vi "Graph_Display.vi"(0 "Data In":T5, 2 "Display State In":T3 {"Time_data" format="%<%.3X>T"}, 3 "Container State":T4) -> (6 "Data Out":T5, 7 "Display State Out":T3 {"Time_data" format="%<%.3X>T"}, 8 "Action":T2)   [LabVIEW 2013, in "2D Buffer Display.xctl"]
doc: "This is the actual display that the user will see when they place the X control on the interface. This display (facade) VI handles user events such as data input and display state changes (i.e. when a control property is updated) as well as an events associated with the actual interface itself (such as scale changes). \nThe 2-D buffer will display a single variable for 0 to n channels where n is specified by the owner of the control. Data in the buffer can be retrieved using properrty nodes as necessary and the amount of data stored in the properrty node can be also adjusted through property nodes."
uses:
  2D Buffer Display.xctl
  Graph_Data.ctl
  <vilib>/_xctls/Container State.ctl
  Graph_State.ctl
  <vilib>/_xctls/Action.ctl
  <vilib>/_xctls/XControlSupport.lvlib
  <vilib>/Analysis/NI_AALBase.lvlib
panel:
  out "Chart":T1(graph)
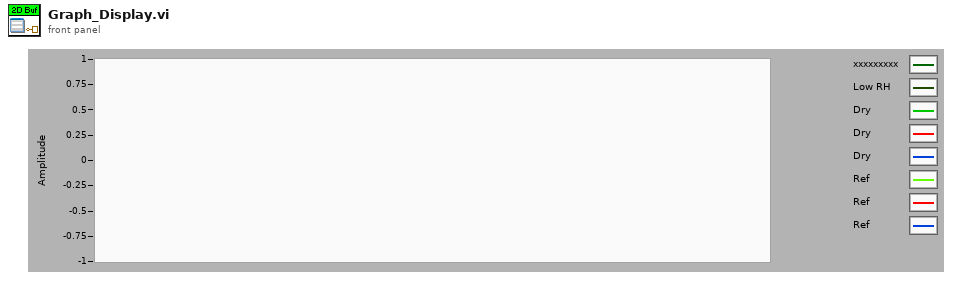
[diagram p1: front panel]
types:
  T1 = cluster{"Time_data":timestamp[], "data_out":sgl[]}[]
  T2 = typedef "XControlSupport.lvlib/Action.ctl" = cluster{"Data Changed?":bool, "State Changed?":bool, "Action Name":string}
  T3 = typedef "2D Buffer Display.xctl/Graph_State.ctl" = cluster{"History":u16, "Time_data":timestamp[], "Data_Out":sgl[][][], "Channels":bool[], "Variable":bool[], "Variable Tags":string[], "Channel Tags":string[], "Plot Details":cluster{"Name":string, "Line Width":u8, "Line Style":u8, "Color":u32}[], "Y-Axis Labels":string[], "Avg Data":cluster{"mean":dbl, "standard deviation":dbl}[][]}
  T4 = typedef "XControlSupport.lvlib/Container State.ctl" = cluster{"Indicator?":bool, "Run Mode?":bool, " Refnum":refnum<vi>}
  T5 = typedef "2D Buffer Display.xctl/Graph_Data.ctl" = cluster{"data_out":sgl[][], "time":timestamp}
  T6 = typedef "LVCursorListTypeDef.ctl" = cluster{"Name":string, "Color":u32, "Style":u8, "Point Style":u8, "Name Visible":bool, "Allow Drag":bool, "Cursor Mode":u32, "Plot":i32, "Index":i32, "Position":cluster{"X":dbl, "Y":dbl}, "X Scale":u32, "Y Scale":u32, "Watch Plots":i32[], "Watch All Plots":bool, "Plot Area":i32, "Label Offset":cluster{"X":dbl, "Y":dbl}}[]
  T7 = cluster{"Name":string, "Line Width":u8, "Line Style":u8, "Color":u32}[]
  T8 = cluster{"Name":string, "Line Width":u8, "Line Style":u8, "Color":u32}
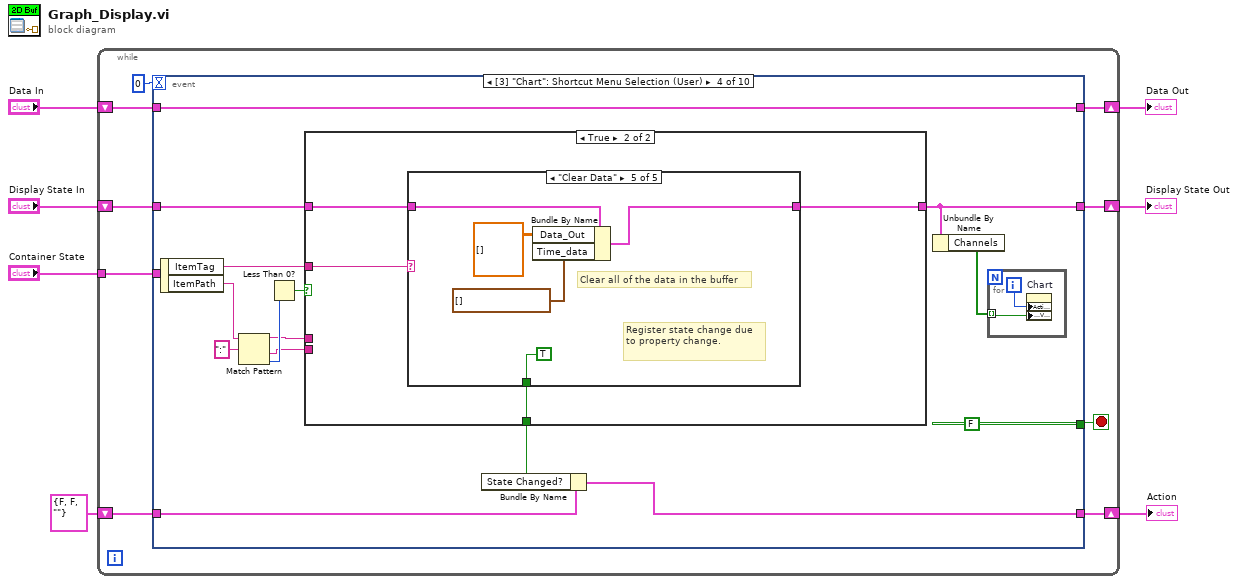
[diagram p0: block diagram]
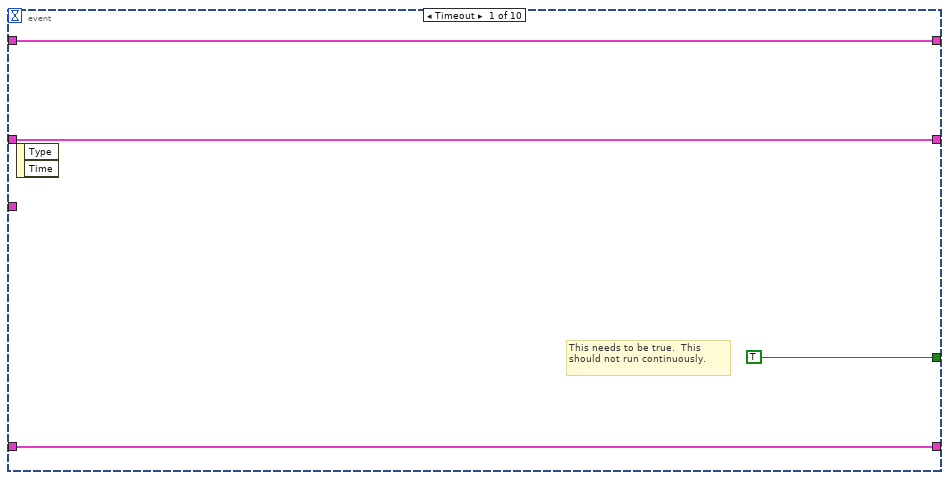
[diagram p2: hidden frame]
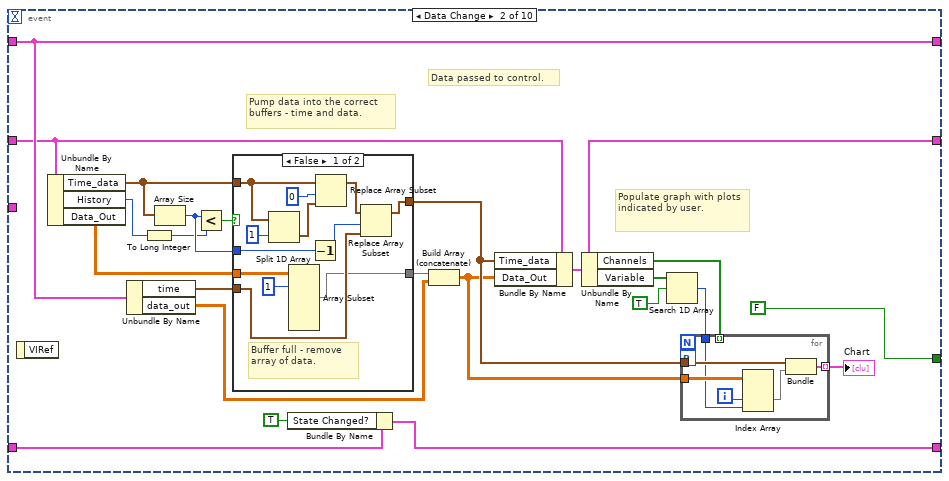
[diagram p3: hidden frame]
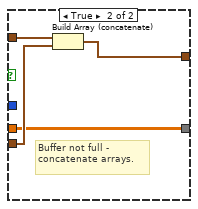
[diagram p4: hidden frame]
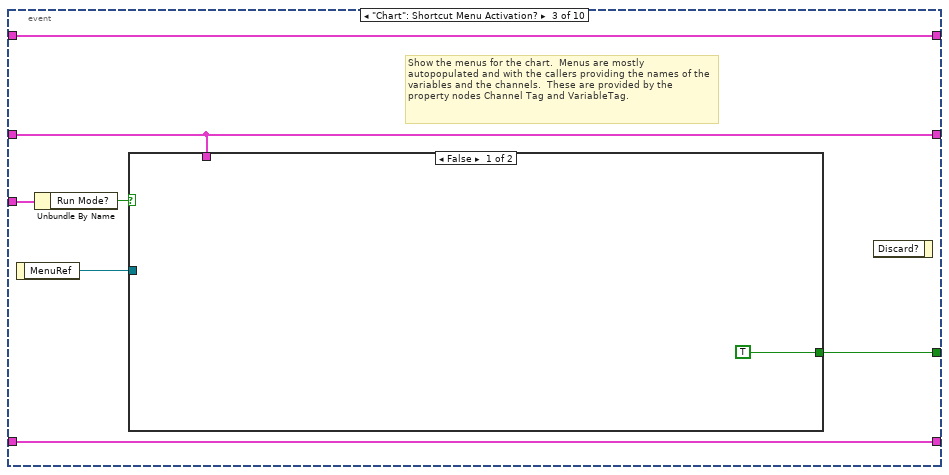
[diagram p5: hidden frame]
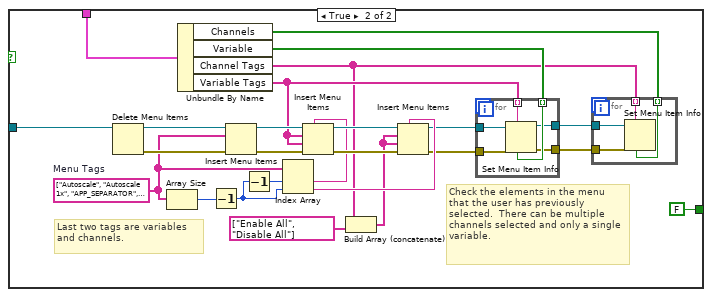
[diagram p6: hidden frame]
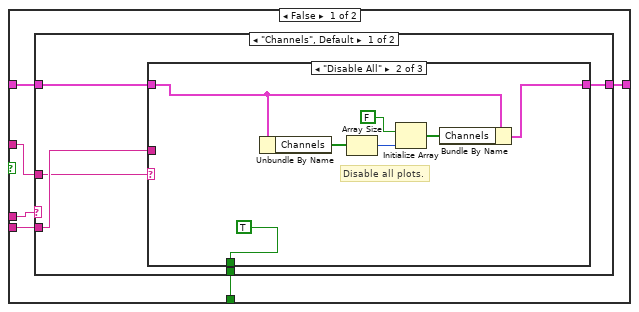
[diagram p7: hidden frame]
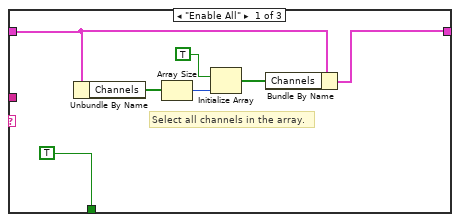
[diagram p8: hidden frame]
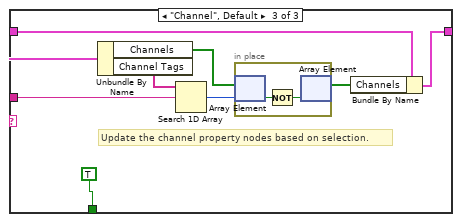
[diagram p9: hidden frame]
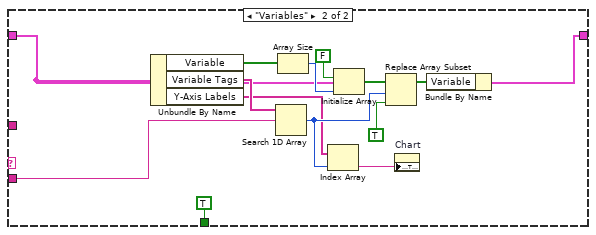
[diagram p10: hidden frame]
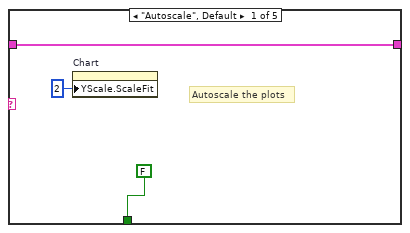
[diagram p11: hidden frame]
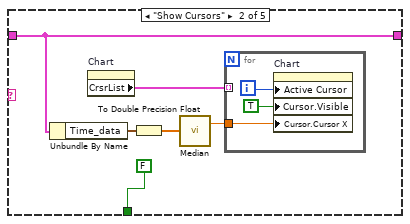
[diagram p12: hidden frame]
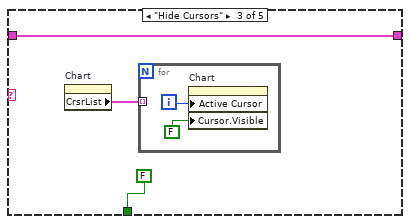
[diagram p13: hidden frame]
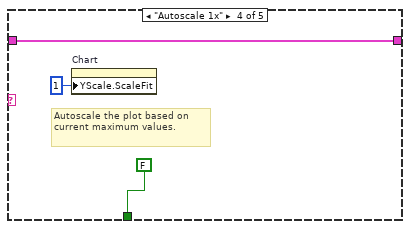
[diagram p14: hidden frame]
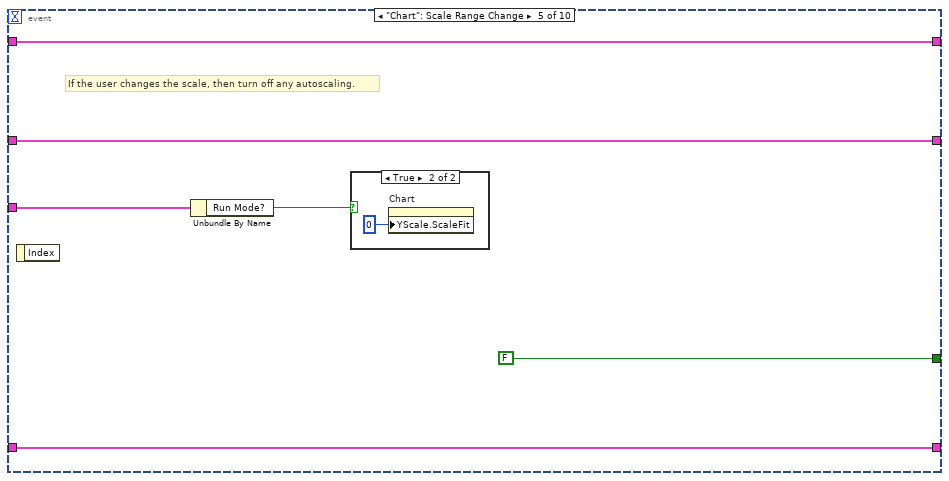
[diagram p15: hidden frame]
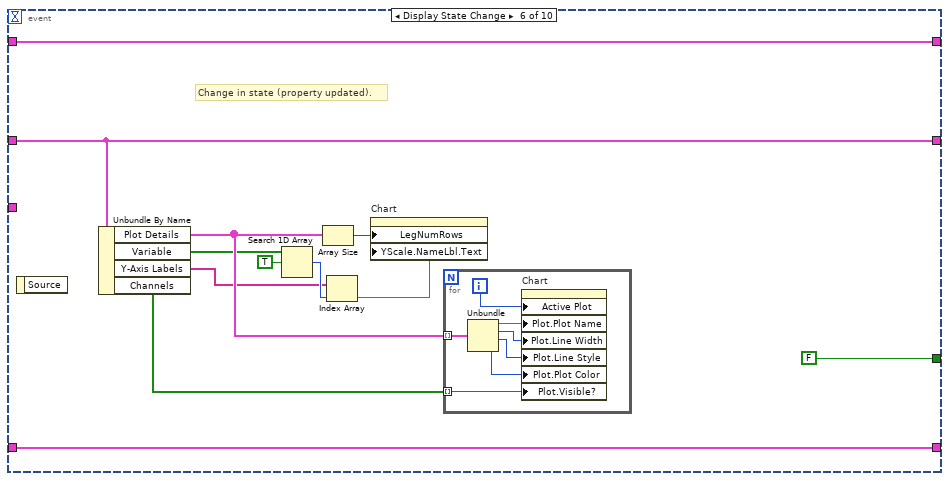
[diagram p17: hidden frame]
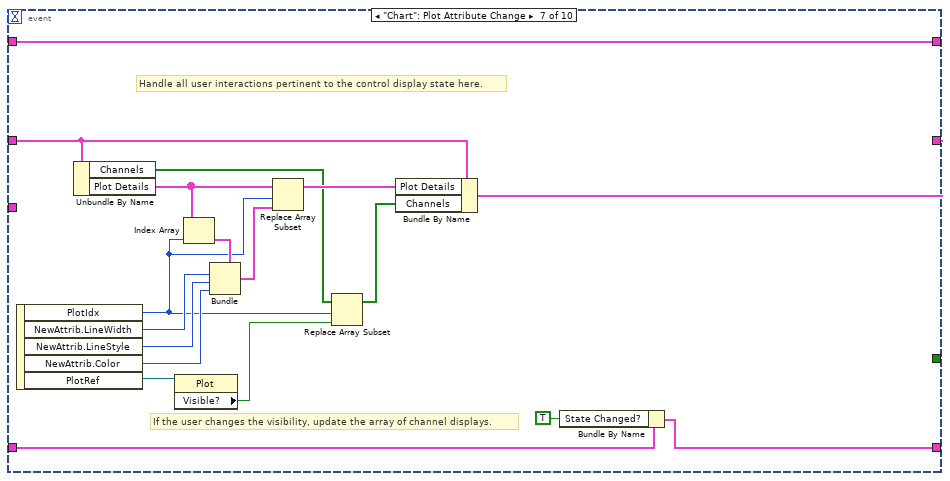
[diagram p18: hidden frame]
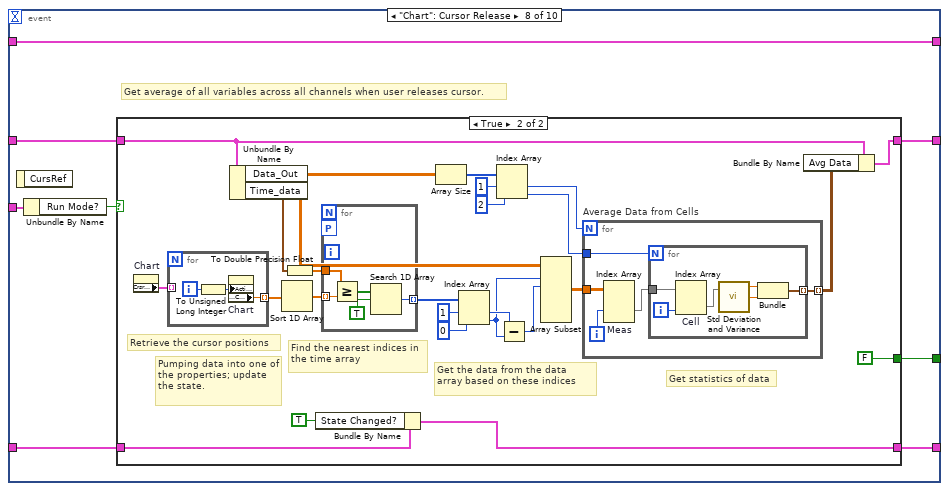
[diagram p19: hidden frame]
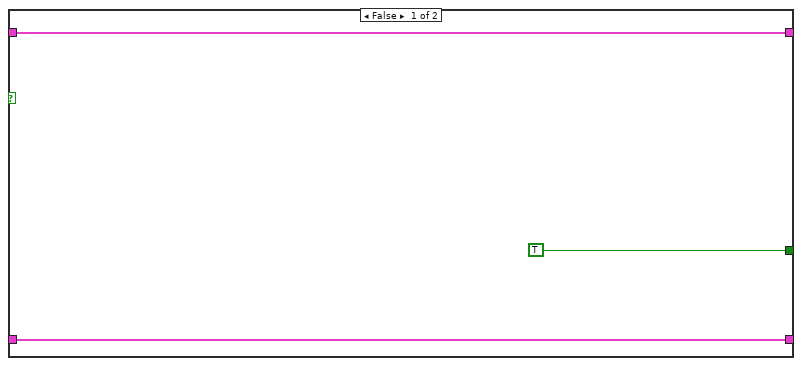
[diagram p20: hidden frame]
diagram:
  n1 = while {
    shift-right: [w15] -> w4
    shift-left: "Display State In" -> [w16]
    tunnel: "Container State" -> [w12]
    shift-right: [w10] -> w7
    shift-left: "Data In" -> [w11]
    shift-right: [w8] -> w2
    shift-left: T2 {"Data Changed?"=FALSE, "State Changed?"=FALSE, "Action Name"=""} ("Action") -> [w9]
    stop <- w14 stop-if-true
    n2 = event shown="[3] \"Chart\": Shortcut Menu Selection (User)" {
      selector: _ -> [_ _ _ _ _ _ _ _ _ _]
      dyn-events: _ -> [_ _ _ _ _ _ _ _ _ _]
      timeout: 0 -> [_ _ _ _ _ _ _ _ _ _]
      tunnel: w16 -> [w18 w40 w69 w118 w208 w217 w246 w254 w306 w310]
      tunnel: [w18 w29 w69 w115 w208 w217 w238 w253 w306 w309] -> w15
      tunnel: [TRUE FALSE w68 FALSE FALSE FALSE _ w250 FALSE FALSE] -> w14
      tunnel: w12 -> [_ _ w67 _ w205 _ _ w249 _ w312]
      tunnel: w11 -> [w17 w41 w72 w123 w209 w222 w247 w255 w305 w314]
      tunnel: [w17 w41 w72 w123 w209 w222 w247 w255 w305 w314] -> w10
      tunnel: [w19 w30 w71 w117 w207 w221 w235 w251 w304 w307] -> w8
      tunnel: w9 -> [w19 w32 w71 w120 w207 w221 w237 w252 w304 w308]
      event Timeout {
        # "This needs to be true.  This should not run continuously."
        n3 = event-data() -> ()  [unwired: 1 in, 2 out]
      }
      event Data Change {
        # "Data passed to control."
        # "Pump data into the correct buffers - time and data."
        # "Populate graph with plots indicated by user."
        n4 = event-data() -> ()  [unwired: 1 in, 1 out]
        n5 = Unbundle By Name(w40) -> ("Time_data"=w43:timestamp[], "History"=w36:u16, "Data_Out"=w39:sgl[][][])
        n6 = Unbundle By Name(w41) -> ("time"=w35:timestamp, "data_out"=w22:sgl[][])
        n7 = To Long Integer(number=w36) -> (32bit integer=w37:i32)
        n8 = Array Size(array=w43) -> (size(s)=w38:i32)
        n9 = Less?(x=w38, y=w37) -> (x < y?=w42:bool)
        n10 = case shown="False" w42 {
          tunnel: w43 -> [w56 w65]
          tunnel: [w55 w63] -> w34
          tunnel: w35 -> [w54 w64]
          tunnel: w39 -> [w51 w62]
          tunnel: w38 -> [w53 _]
          tunnel: [w50 w62] -> w24
          frame False {
            # "Buffer full - remove array of data."
            n11 = Split 1D Array(array=w56, index=1) -> (second subarray=w57:timestamp[])  [unwired: 1 out]
            n12 = Array Subset(array=w51, index (dim 0)=1 ("index")) -> (w50:sgl[][][])  [unwired: 5 in]
            n13 = Decrement(x=w53) -> (x-1=w59:i32)
            n14 = Replace Array Subset(array=w56, new element=w57, index=0) -> (w60:timestamp[])
            n15 = Replace Array Subset(array=w60, new element=w54, index=w59) -> (w55:timestamp[])
          }
          frame True {
            # "Buffer not full - concatenate arrays."
            n16 = Build Array (concatenate)(w65, w64) -> (w63:timestamp[])
          }
        }
        n17 = Bundle By Name(cluster=w32, "State Changed?"=TRUE) -> (w30:T2)
        n18 = Build Array (concatenate)(w24, w22) -> (w23:sgl[][][])
        n19 = Bundle By Name(cluster=w40, "Time_data"=w34, "Data_Out"=w23) -> (w29:T3)
        n20 = Unbundle By Name(w29) -> ("Channels"=w25:bool[], "Variable"=w28:bool[])
        n21 = Search 1D Array(1D array=w28, element=TRUE) -> (index of element=w26:i32)  [unwired: 1 in]
        n22 = for {
          tunnel: w34 -> [w49]
          tunnel: w23 -> [w48]
          tunnel: w26 -> [w47]
          tunnel: w25 -> [_] mode=indexing
          tunnel: [w44] -> w21 mode=indexing
          workers-P: _ -> [_]
          i -> [w46]
          n23 = Index Array(array=w48, index (dim 1)=w46, index (dim 2)=w47) -> (element=w45:sgl[])  [unwired: 1 in]
          n24 = Bundle("Time_data"=w49, w45) -> (w44:cluster{"Time_data":timestamp[], sgl[]})  [unwired: 1 in]
        }
        "Chart" <- w21
      }
      event "Chart": Shortcut Menu Activation? {
        # "Show the menus for the chart.  Menus are mostly autopopulated and with the callers providing the names of the variables and the channels.  These are provided by the property nodes Channel Tag and VariableTag."
        n25 = event-data() -> ("MenuRef"=w70:refnum<k9>)  [unwired: 1 in]
        n26 = Unbundle By Name(w67) -> ("Run Mode?"=w66:bool)
        n27 = case shown="False" w66 {
          tunnel: w70 -> [_ w98]
          tunnel: w69 -> [_ w91]
          tunnel: [TRUE FALSE] -> w68
          frame False {
          }
          frame True {
            w77 = string[] ["Autoscale", "Autoscale 1x", "APP_SEPARATOR", "Show Cursors", "Hide Cursors", "Clear Data", "APP_SEPARATOR", "Variables", "Channels"]  # Menu Tags
            # "Check the elements in the menu that the user has previously selected.  There can be multiple channels selected and only a single variable."
            # "Last two tags are variables and channels."
            n28 = Delete Menu Items(9:w98) -> (0:w96:errorcluster, 3:w97:refnum<k9>)  [unwired: 3 in]
            n29 = Array Size(array=w77) -> (size(s)=w76:i32)
            n30 = Unbundle By Name(w91) -> ("Channels"=w84:bool[], "Variable"=w86:bool[], "Channel Tags"=w80:string[], "Variable Tags"=w85:string[])
            n31 = Decrement(x=w76) -> (x-1=w74:i32)
            n32 = Insert Menu Items(6:w96, 8:w77, 9:w97) -> (0:w94:errorcluster, 3:w95:refnum<k9>)  [unwired: 3 in, 1 out]
            n33 = Decrement(x=w74) -> (x-1=w75:i32)
            n34 = Index Array(array=w77, index #1=w75, index #2=w74) -> (element #1=w90:string, element #2=w89:string)
            n35 = Insert Menu Items(5:w90, 6:w94, 7:w85, 8:w85, 9:w95) -> (0:w92:errorcluster, 3:w93:refnum<k9>)  [unwired: 1 in, 1 out]
            n36 = Build Array (concatenate)(w80, string[] ["Enable All", "Disable All"]) -> (w78:string[])
            n37 = Insert Menu Items(5:w89, 6:w92, 7:w78, 8:w78, 9:w93) -> (0:w88:errorcluster, 3:w87:refnum<k9>)  [unwired: 1 in, 1 out]
            n38 = for {
              tunnel: w88 -> [w108]
              tunnel: w87 -> [w107]
              tunnel: w86 -> [w106] mode=indexing
              tunnel: w85 -> [w103] mode=indexing
              tunnel: [w105] -> w83
              tunnel: [w104] -> w82
              n39 = Set Menu Item Info(6:w106, 7:w103, 8:w108, 11:w107) -> (0:w104:errorcluster, 3:w105:refnum<k9>)  [unwired: 3 in]
            }
            n40 = for {
              tunnel: w82 -> [w102]
              tunnel: w83 -> [w101]
              tunnel: w84 -> [w100] mode=indexing
              tunnel: w80 -> [w99] mode=indexing
              n41 = Set Menu Item Info(6:w100, 7:w99, 8:w102, 11:w101) -> ()  [unwired: 3 in, 2 out]
            }
          }
        }
        n42 = event-data() -> ()  [unwired: 2 in, 1 out]
      }
      event "Chart": Shortcut Menu Selection (User) {
        n43 = event-data() -> ("ItemTag"=w121:string, "ItemPath"=w111:string)  [unwired: 1 in]
        n44 = Match Pattern(string=w111, regular expression=":" ("search string/char (-)")) -> (before substring=w112:string, after substring=w109:string, offset past match=w113:i32)  [unwired: 1 in, 1 out]
        n45 = Less Than 0?(x=w113) -> (x < 0?=w122:bool)
        n46 = case shown="True" w122 {
          tunnel: w121 -> [w126 w178]
          tunnel: [w130 w177] -> w119
          tunnel: w118 -> [w131 w176]
          tunnel: [w129 w175] -> w115
          tunnel: w112 -> [w128 _]
          tunnel: w109 -> [w127 _]
          frame False {
            n47 = case shown="\"Channels\", Default" w128 {
              tunnel: w131 -> [w136 w164]
              tunnel: [w134 TRUE] -> w130
              tunnel: [w135 w162] -> w129
              tunnel: w127 -> [w133 w163]
              tunnel: w126 -> [w132 _]
              frame "Channels", Default {
                n48 = case shown="\"Disable All\"" w132 {
                  tunnel: w136 -> [w138 w146 w158]
                  tunnel: [w137 w145 w157] -> w135
                  tunnel: [TRUE TRUE TRUE] -> w134
                  tunnel: w133 -> [_ _ w151]
                  frame "Enable All" {
                    # "Select all channels in the array."
                    n49 = Unbundle By Name(w138) -> ("Channels"=w140:bool[])
                    n50 = Array Size(array=w140) -> (size(s)=w143:i32)
                    n51 = Initialize Array(TRUE, w143) -> (w141:bool[])
                    n52 = Bundle By Name(cluster=w138, "Channels"=w141) -> (w137:T3)
                  }
                  frame "Disable All" {
                    # "Disable all plots."
                    n53 = Unbundle By Name(w146) -> ("Channels"=w147:bool[])
                    n54 = Array Size(array=w147) -> (size(s)=w150:i32)
                    n55 = Initialize Array(FALSE, w150) -> (w148:bool[])
                    n56 = Bundle By Name(cluster=w146, "Channels"=w148) -> (w145:T3)
                  }
                  frame "Channel", Default {
                    # "Update the channel property nodes based on selection."
                    n57 = Unbundle By Name(w158) -> ("Channels"=w154:bool[], "Channel Tags"=w155:string[])
                    n58 = Search 1D Array(1D array=w155, element=w151) -> (index of element=w153:i32)  [unwired: 1 in]
                    n59 = in-place {
                      n60 = in-place-array #1(w154, w153) -> (w160:bool)
                      n61 = Not(x=w160) -> (.not. x?=w159:bool)
                      n62 = in-place-array #1(w159) -> (w152:bool[])  [unwired: 1 out]
                    }
                    n63 = Bundle By Name(cluster=w158, "Channels"=w152) -> (w157:T3)
                  }
                }
              }
              frame "Variables" {
                n64 = Unbundle By Name(w164) -> ("Variable"=w173:bool[], "Variable Tags"=w174:string[], "Y-Axis Labels"=w166:string[])
                n65 = Search 1D Array(1D array=w174, element=w163) -> (index of element=w167:i32)  [unwired: 1 in]
                n66 = Array Size(array=w173) -> (size(s)=w172:i32)
                n67 = Index Array(array=w166, index=w167) -> (element=w165:string)
                n68 = Initialize Array(FALSE, w172) -> (w170:bool[])
                n69 = Replace Array Subset(array=w170, new element=TRUE ("new element/subarray"), index=w167) -> (w168:bool[])
                n70 = property on="Chart" class="XYGraph (strict)"("YScale.NameLbl.Text"=w165) -> ()  [unwired: 2 in, 2 out]
                n71 = Bundle By Name(cluster=w164, "Variable"=w168) -> (w162:T3)
              }
            }
          }
          frame True {
            n72 = case shown="\"Clear Data\"" w178 {
              tunnel: [FALSE FALSE FALSE FALSE TRUE] -> w177
              tunnel: w176 -> [w179 w185 w193 w196 w202]
              tunnel: [w179 w185 w193 w196 w199] -> w175
              frame "Autoscale", Default {
                # "Autoscale the plots"
                n73 = property on="Chart" class="XYGraph (strict)"("YScale.ScaleFit"=u8 2 ("Y Scale.Scale Fit")) -> ()  [unwired: 2 in, 2 out]
              }
              frame "Show Cursors" {
                n74 = Unbundle By Name(w185) -> ("Time_data"=w184:timestamp[])
                n75 = property on="Chart" class="XYGraph (strict)"() -> ("CrsrList"=w187:T6)  [unwired: 2 in, 2 out]
                n76 = To Double Precision Float(number=w184) -> (double precision float=w183:dbl[])
                n77 = call <vilib>:"Median.vi"("X"=w183) -> ("median"=w182:dbl)  [unwired: 1 out]
                n78 = for {
                  tunnel: w187 -> [_] mode=indexing
                  tunnel: w182 -> [w188]
                  i -> [w190]
                  n79 = property on="Chart" class="XYGraph (strict)"("Active Cursor"=w190, "Cursor.Visible"=TRUE, "Cursor.Cursor X"=w188) -> ()  [unwired: 2 in, 2 out]
                }
              }
              frame "Hide Cursors" {
                n80 = property on="Chart" class="XYGraph (strict)"() -> ("CrsrList"=w192:T6)  [unwired: 2 in, 2 out]
                n81 = for {
                  tunnel: w192 -> [_] mode=indexing
                  i -> [w195]
                  n82 = property on="Chart" class="XYGraph (strict)"("Active Cursor"=w195, "Cursor.Visible"=FALSE) -> ()  [unwired: 2 in, 2 out]
                }
              }
              frame "Autoscale 1x" {
                # "Autoscale the plot based on current maximum values."
                n83 = property on="Chart" class="XYGraph (strict)"("YScale.ScaleFit"=u8 1 ("Y Scale.Scale Fit")) -> ()  [unwired: 2 in, 2 out]
              }
              frame "Clear Data" {
                # "Register state change due to property change."
                # "Clear all of the data in the buffer"
                n84 = Bundle By Name(cluster=w202, "Data_Out"=sgl[][][] [], "Time_data"=timestamp[] []) -> (w199:T3)
              }
            }
          }
        }
        n85 = Bundle By Name(cluster=w120, "State Changed?"=w119) -> (w117:T2)
        n86 = Unbundle By Name(w115) -> ("Channels"=w114:bool[])
        n87 = for {
          tunnel: w114 -> [w124] mode=indexing
          i -> [w125]
          n88 = property on="Chart" class="XYGraph (strict)"("Active Plot"=w125, "Plot.Visible?"=w124) -> ()  [unwired: 2 in, 2 out]
        }
      }
      event "Chart": Scale Range Change {
        # "If the user changes the scale, then turn off any autoscaling."
        n89 = event-data() -> ()  [unwired: 1 in, 1 out]
        n90 = Unbundle By Name(w205) -> ("Run Mode?"=w204:bool)
        n91 = case shown="True" w204 {
          frame False {
          }
          frame True {
            n92 = property on="Chart" class="XYGraph (strict)"("YScale.ScaleFit"=u8 0 ("Y Scale.Scale Fit")) -> ()  [unwired: 2 in, 2 out]
          }
        }
      }
      event Display State Change {
        # "Change in state (property updated)."
        n93 = event-data() -> ()  [unwired: 1 in, 1 out]
        n94 = Unbundle By Name(w217) -> ("Plot Details"=w218:T7, "Variable"=w216:bool[], "Y-Axis Labels"=w213:string[], "Channels"=w211:bool[])
        n95 = Search 1D Array(1D array=w216, element=TRUE) -> (index of element=w214:i32)  [unwired: 1 in]
        n96 = Array Size(array=w218) -> (size(s)=w219:i32)
        n97 = Index Array(array=w213, index=w214) -> (element=w212:string)
        n98 = property on="Chart" class="XYGraph (strict)"("LegNumRows"=w219, "YScale.NameLbl.Text"=w212) -> ()  [unwired: 2 in, 2 out]
        n99 = for {
          tunnel: w218 -> [w228] mode=indexing
          tunnel: w211 -> [w223] mode=indexing
          i -> [w229]
          n100 = Unbundle(w228) -> ("Name"=w227:string, "Line Width"=w226:u8, "Line Style"=w225:u8, "Color"=w224:u32)
          n101 = property on="Chart" class="XYGraph (strict)"("Active Plot"=w229, "Plot.Plot Name"=w227, "Plot.Line Width"=w226, "Plot.Line Style"=w225, "Plot.Plot Color"=w224, "Plot.Visible?"=w223) -> ()  [unwired: 2 in, 2 out]
        }
      }
      event "Chart": Plot Attribute Change {
        # "If the user changes the visibility, update the array of channel displays."
        # "Handle all user interactions pertinent to the control display state here."
        n102 = event-data() -> ("PlotIdx"=w233:i32, "NewAttrib.LineWidth"=w242:u8, "NewAttrib.LineStyle"=w243:u8, "NewAttrib.Color"=w244:u32, "PlotRef"=w234:refnum<vi>)  [unwired: 1 in]
        n103 = Unbundle By Name(w246) -> ("Channels"=w230:bool[], "Plot Details"=w241:T7)
        n104 = property class="Plot"(reference=w234) -> ("Visible?"=w232:bool)  [unwired: 1 in, 2 out]
        n105 = Index Array(array=w241, index=w233) -> (element=w245:T8)
        n106 = Bundle(cluster=w245, "Line Width"=w242, "Line Style"=w243, "Color"=w244) -> (w240:T8)  [unwired: 1 in]
        n107 = Replace Array Subset(array=w241, new element=w240, index=w233) -> (w239:T7)
        n108 = Replace Array Subset(array=w230, new element=w232, index=w233) -> (w231:bool[])
        n109 = Bundle By Name(cluster=w246, "Plot Details"=w239, "Channels"=w231) -> (w238:T3)
        n110 = Bundle By Name(cluster=w237, "State Changed?"=TRUE) -> (w235:T2)
      }
      event "Chart": Cursor Release {
        # "Get average of all variables across all channels when user releases cursor."
        n111 = event-data() -> ()  [unwired: 1 in, 1 out]
        n112 = Unbundle By Name(w249) -> ("Run Mode?"=w248:bool)
        n113 = case shown="True" w248 {
          tunnel: w254 -> [w258 w265]
          tunnel: [w258 w263] -> w253
          tunnel: w252 -> [w257 w262]
          tunnel: [w257 w260] -> w251
          tunnel: [TRUE FALSE] -> w250
          frame False {
          }
          frame True {
            # "Pumping data into one of the properties; update the state."
            # "Get statistics of data"
            # "Get the data from the data array based on these indices"
            # "Find the nearest indices in the time array"
            # "Retrieve the cursor positions"
            n114 = property on="Chart" class="XYGraph (strict)"() -> ("CrsrList"=w283:T6)  [unwired: 2 in, 2 out]
            n115 = for {
              tunnel: w283 -> [_] mode=indexing
              tunnel: [w302] -> w281 mode=indexing
              i -> [w300]
              n116 = To Unsigned Long Integer(number=w300) -> (unsigned 32bit integer=w301:u32)
              n117 = property on="Chart" class="XYGraph (strict)"("Active Cursor"=w301) -> ("Cursor.Cursor X"=w302:dbl)  [unwired: 2 in, 2 out]
            }
            n118 = Unbundle By Name(w265) -> ("Data_Out"=w271:sgl[][][], "Time_data"=w282:timestamp[])
            n119 = Sort 1D Array(array=w281) -> (sorted array=w279:dbl[])
            n120 = To Double Precision Float(number=w282) -> (double precision float=w280:dbl[])
            n121 = Bundle By Name(cluster=w262, "State Changed?"=TRUE) -> (w260:T2)
            n122 = for {
              tunnel: w280 -> [w299]
              tunnel: w279 -> [w298] mode=indexing
              tunnel: [w295] -> w278 mode=indexing
              workers-P: _ -> [_]
              n123 = Greater Or Equal?(x=w299, y=w298) -> (x >= y?=w297:bool[])
              n124 = Search 1D Array(1D array=w297, element=TRUE) -> (index of element=w295:i32)  [unwired: 1 in]
            }
            n125 = Array Size(array=w271) -> (size(s)=w270:i32[])
            n126 = Index Array(array=w278, index #1=1 ("index"), index #2=0 ("index")) -> (element #1=w275:i32, element #2=w274:i32)
            n127 = Index Array(array=w270, index #1=1 ("index"), index #2=2 ("index")) -> (element #1=w269:i32, element #2=w268:i32)
            n128 = Subtract(x=w275, y=w274) -> (x-y=w273:i32)
            n129 = Array Subset(array=w271, index (dim 0)=w274, length (dim 0)=w273) -> (w272:sgl[][][])  [unwired: 4 in]
            n130 = for "Average Data from Cells" {
              N: w269 -> [_]
              tunnel: w272 -> [w287]
              tunnel: [w288] -> w264 mode=indexing
              tunnel: w268 -> [w284]
              i -> [w286]
              n131 = Index Array "Meas"(array=w287, index (dim 1)=w286) -> (element=w285:sgl[][])  [unwired: 2 in]
              n132 = for {
                N: w284 -> [_]
                tunnel: w285 -> [w291]
                tunnel: [w292] -> w288 mode=indexing
                i -> [w290]
                n133 = Index Array "Cell"(array=w291, index (col)=w290) -> (element=w289:sgl[])  [unwired: 1 in]
                n134 = call <vilib>:"Std Deviation and Variance.vi"("X"=w289) -> ("mean"=w294:dbl, "standard deviation"=w293:dbl)  [unwired: 1 in, 1 out]
                n135 = Bundle("mean"=w294, "standard deviation"=w293) -> (w292:cluster{"mean":dbl, "standard deviation":dbl})  [unwired: 1 in]
              }
            }
            n136 = Bundle By Name(cluster=w265, "Avg Data"=w264) -> (w263:T3)
          }
        }
      }
      event Direction Change {
        # "Change from indicator to control or vice-versa."
        n137 = event-data() -> ()  [unwired: 1 in, 1 out]
      }
      event Exec State Change {
        # "Indicates change from edit to run mode."
        n138 = event-data() -> ()  [unwired: 1 in, 1 out]
        n139 = Unbundle By Name(w312) -> ("Run Mode?"=w311:bool)
        n140 = case shown="True" w311 {
          tunnel: w310 -> [w316 w326]
          tunnel: [w316 w319] -> w309
          tunnel: w308 -> [w315 w322]
          tunnel: [w315 w320] -> w307
          frame False {
          }
          frame True {
            # "Clear the plot when we got to run mode"
            n141 = Bundle By Name(cluster=w326, "History"=u16 300, "Time_data"=timestamp[] [], "Data_Out"=sgl[][][] []) -> (w319:T3)
            n142 = Bundle By Name(cluster=w322, "State Changed?"=TRUE) -> (w320:T2)
            n143 = Unbundle By Name(w319) -> ("Plot Details"=w318:T7)
            n144 = Array Size(array=w318) -> (size(s)=w317:i32)
            n145 = for {
              tunnel: w318 -> [w331] mode=indexing
              i -> [w332]
              n146 = Unbundle(w331) -> ("Name"=w330:string, "Line Width"=w329:u8, "Line Style"=w328:u8, "Color"=w327:u32)
              n147 = property on="Chart" class="XYGraph (strict)"("Active Plot"=w332, "Plot.Plot Name"=w330, "Plot.Line Width"=w329, "Plot.Line Style"=w328, "Plot.Plot Color"=w327) -> ()  [unwired: 2 in, 2 out]
            }
            n148 = property on="Chart" class="XYGraph (strict)"("LegNumRows"=w317) -> ()  [unwired: 2 in, 2 out]
          }
        }
      }
    }
  }
  "Display State Out" <- w4
  "Data Out" <- w7
  "Action" <- w2
